vi "ReadFlow Example.vi"() -> ()   [LabVIEW 2012]
uses:
  BrooksDLL.dll
panel:
  out "S2 String":string
  out "S1 String":string
  out "S2":u8 format="%.0x"
  out "S1":u8 format="%.0x"
  out "Function Output Comment":string
  out "Flow Unit String":string
  out "Flow Units":u8
  out "Flow":sgl format="%.2f"
  out "output param":i32
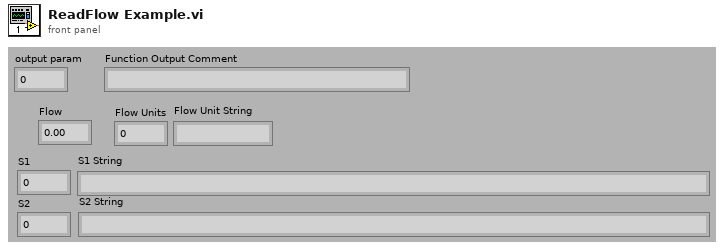
[diagram p1: front panel]
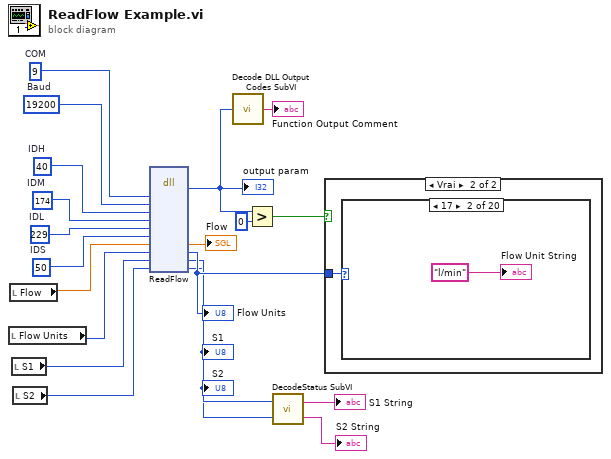
[diagram p0: block diagram]
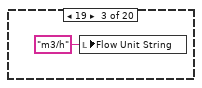
[diagram p4: hidden frame]
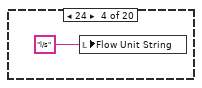
[diagram p5: hidden frame]
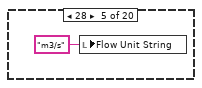
[diagram p6: hidden frame]
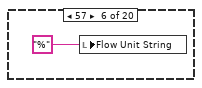
[diagram p7: hidden frame]
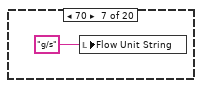
[diagram p8: hidden frame]
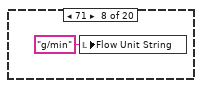
[diagram p9: hidden frame]
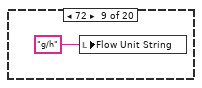
[diagram p10: hidden frame]
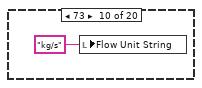
[diagram p11: hidden frame]
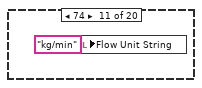
[diagram p12: hidden frame]
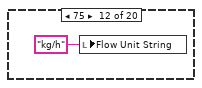
[diagram p13: hidden frame]
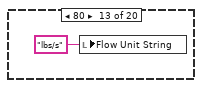
[diagram p14: hidden frame]
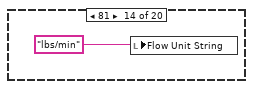
[diagram p15: hidden frame]
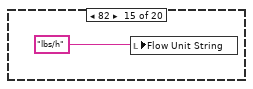
[diagram p16: hidden frame]
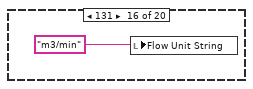
[diagram p17: hidden frame]
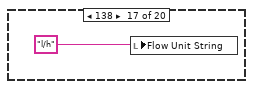
[diagram p18: hidden frame]
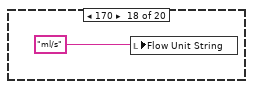
[diagram p19: hidden frame]
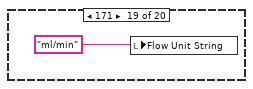
[diagram p20: hidden frame]
diagram:
  w15 = u8 50  # IDS
  w16 = u8 229  # IDL
  w17 = u8 174  # IDM
  w18 = u8 40  # IDH
  w19 = 19200  # Baud
  w20 = 9  # COM
  n1 = local read "Flow Units"() -> (w10:u8)
  n2 = local read "Flow"() -> (w7:sgl)
  n3 = local read "S1"() -> (w6:u8)
  n4 = local read "S2"() -> (w5:u8)
  n5 = dll-call lib="C:/Users/Sylvain/Desktop/TopPerm_20150127/drivers/Brooks/S Protocol/BrooksDLL.dll" fn="ReadFlow"("COM"=w20, "Baud"=w19, "IDH"=w18, "IDM"=w17, "IDL"=w16, "IDS"=w15, "Flow"=w7, "FlowUnit"=w10, "S1"=w6, "S2"=w5) -> (w12:i32, "Flow"=→"Flow":sgl, "FlowUnit"=w9:u8, "S1"=w4:u8, "S2"=w3:u8)  [unwired: 9 in, 2 out]
  "output param" <- w12
  "Flow Units" <- w9
  "S1" <- w4
  "S2" <- w3
  n6 = call "Decode DLL Output Codes SubVI.vi"("Numeric"=w12) -> ("Function Output Comment"=→"Function Output Comment":string)
  n7 = Greater?(x=w12, y=0) -> (0:w14:bool)
  n8 = call "DecodeStatus SubVI.vi"("S2"=w3, "S1"=w4) -> ("S2 String"=→"S2 String":string, "S1 String"=→"S1 String":string)
  n9 = case shown="Vrai" w14 {
    tunnel: w9 -> [_ w21]
    frame False {
    }
    frame True {
      n10 = case shown="17" w21 {
        frame 0, Default {
        }
        frame 17 {
          "Flow Unit String" <- "l/min"
        }
        frame 19 {
          n11 = local write "Flow Unit String"("m3/h") -> ()
        }
        frame 24 {
          n12 = local write "Flow Unit String"("l/s") -> ()
        }
        frame 28 {
          n13 = local write "Flow Unit String"("m3/s") -> ()
        }
        frame 57 {
          n14 = local write "Flow Unit String"("%") -> ()
        }
        frame 70 {
          n15 = local write "Flow Unit String"("g/s") -> ()
        }
        frame 71 {
          n16 = local write "Flow Unit String"("g/min") -> ()
        }
        frame 72 {
          n17 = local write "Flow Unit String"("g/h") -> ()
        }
        frame 73 {
          n18 = local write "Flow Unit String"("kg/s") -> ()
        }
        frame 74 {
          n19 = local write "Flow Unit String"("kg/min") -> ()
        }
        frame 75 {
          n20 = local write "Flow Unit String"("kg/h") -> ()
        }
        frame 80 {
          n21 = local write "Flow Unit String"("lbs/s") -> ()
        }
        frame 81 {
          n22 = local write "Flow Unit String"("lbs/min") -> ()
        }
        frame 82 {
          n23 = local write "Flow Unit String"("lbs/h") -> ()
        }
        frame 131 {
          n24 = local write "Flow Unit String"("m3/min") -> ()
        }
        frame 138 {
          n25 = local write "Flow Unit String"("l/h") -> ()
        }
        frame 170 {
          n26 = local write "Flow Unit String"("ml/s") -> ()
        }
        frame 171 {
          n27 = local write "Flow Unit String"("ml/min") -> ()
        }
        frame 172 {
          n28 = local write "Flow Unit String"("ml/h") -> ()
        }
      }
    }
  }
